vi "Check Packet ID Unused.vi"(8 "error in (no error)":errorcluster, 10 "PUBLISH":refnum<class "PUBLISH.lvclass">, 11 "Subscription in":refnum<class "Subscription.lvclass">) -> (0 "error out":errorcluster, 2 "PUBLISH out":refnum<class "PUBLISH.lvclass">, 3 "Subscription out":refnum<class "Subscription.lvclass">)   [LabVIEW 2013, in "MQTT Server.lvlib" / "Subscription.lvclass"]
uses:
  Subscription.lvclass
  <vilib>/LabVIEW Open Source Project/MQTT Control Packets/Control Packets/PUBLISH/PUBLISH.lvclass
  Subscription.lvclass/Subscription.ctl
  <vilib>/LabVIEW Open Source Project/MQTT Control Packets/Control Packets/ControlPacket/ControlPacket.lvclass/ControlPacket.ctl
  Stored Packet -- cluster.ctl
  <vilib>/LabVIEW Open Source Project/MQTT Control Packets/Control Packets/ControlPacket/ControlPacket.lvclass
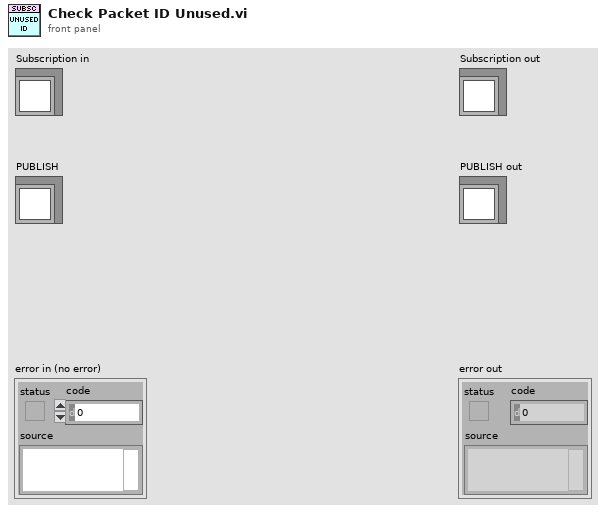
[diagram p1: front panel]
types:
  T1 = typedef "MQTT Server.lvlib/Subscription.lvclass/Stored Packet -- cluster.ctl" = cluster{"Packet Identifier":u16, "ControlPacket":refnum<class "ControlPacket.lvclass">, "last attempt":timestamp}
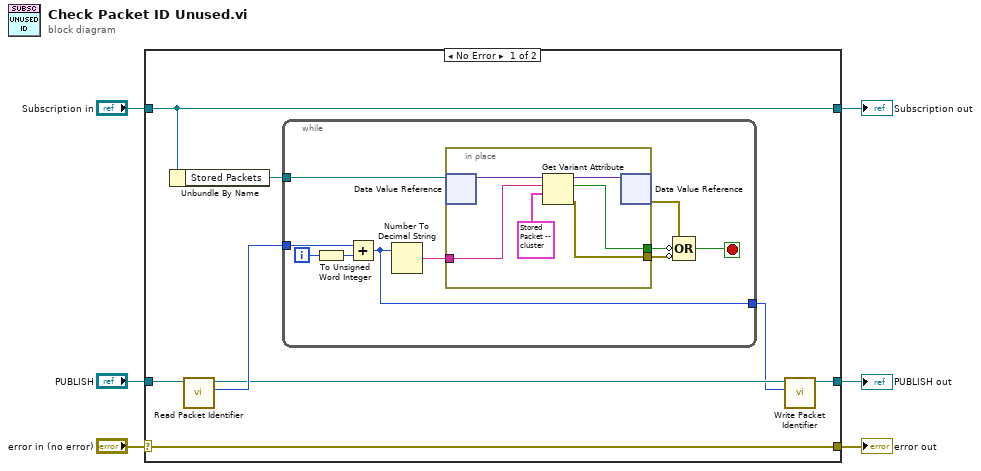
[diagram p0: block diagram]
diagram:
  n1 = case shown="No Error" "error in (no error)" {
    selector: "error in (no error)" -> [w14 w33]
    tunnel: [w14 w33] -> w5
    tunnel: [w13 w32] -> w3
    tunnel: "Subscription in" -> [w13 w32]
    tunnel: "PUBLISH" -> [w11 w31]
    tunnel: [w7 w31] -> w1
    frame No Error {
      n2 = Unbundle By Name(w13) -> ("Stored Packets"=w12:refnum<data-value>)
      n3 = call <vilib>:"Read Packet Identifier.vi"("ControlPacket in"=w11) -> ("Packet Identifier"=w10:u16, "ControlPacket out"=w9:refnum<class "PUBLISH.lvclass">)  [unwired: 9 in]
      n4 = while {
        tunnel: w12 -> [w24]
        tunnel: w10 -> [w17]
        tunnel: [w16] -> w8
        i -> [w18]
        stop <- w19 stop-if-true
        n5 = To Unsigned Word Integer(number=w18) -> (unsigned 16bit integer=w15:u16)
        n6 = Add(x=w17, y=w15) -> (x+y=w16:u16)
        n7 = Number To Decimal String(number=w16) -> (decimal integer string=w23:string)  [unwired: 1 in]
        n8 = in-place {
          in-place-border: w23 -> [w28]
          in-place-border: [w27] -> w21
          in-place-border: [w26] -> w20
          n9 = in-place-dvr #1(w24) -> (w30:variant)  [unwired: 1 out]
          n10 = Get Variant Attribute(Variant=w30, name=w28, default value (empty Variant)=T1 {"Packet Identifier"=0, "ControlPacket"=refnum, "last attempt"=timestamp(0 s since 1904-01-01)} ("Stored Packet")) -> (duplicate Variant=w29:variant, found=w27:bool, error out=w26:errorcluster)  [unwired: 1 in, 1 out]
          n11 = in-place-dvr #1(w29) -> (w22:errorcluster)  [unwired: 1 out]
        }
        n12 = Compound Arithmetic op=OR(w22, invert w21, invert w20) -> (w19:bool)
      }
      n13 = call <vilib>:"Write Packet Identifier.vi"("Packet Identifier"=w8, "ControlPacket in"=w9) -> ("ControlPacket out"=w7:refnum<class "PUBLISH.lvclass">)  [unwired: 9 in]
    }
    frame Error {
    }
  }
  "error out" <- w5
  "Subscription out" <- w3
  "PUBLISH out" <- w1
